vi "getTestTime.vi"(8 "错误输入（无错误）":errorcluster, 11 "startTime":string) -> (0 "错误输出":errorcluster, 3 "timeArray":string[](array[string]))   [LabVIEW 2011]
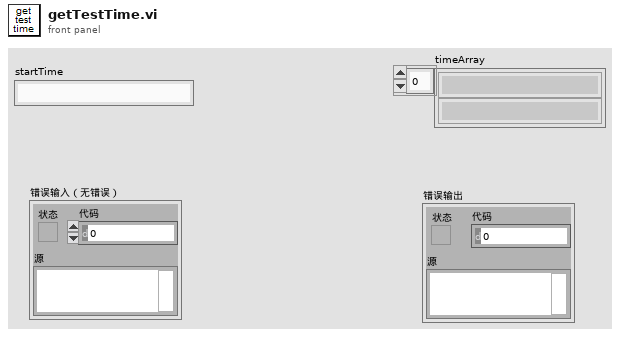
[diagram p1: front panel]
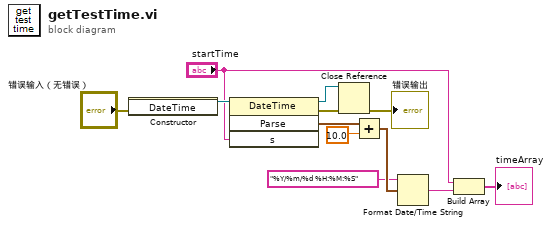
[diagram p0: block diagram]
diagram:
  n1 = constructor class="DateTime"(error in="错误输入（无错误）") -> (reference out=w12:refnum<k24>)  [unwired: 2 in, 2 out]
  n2 = invoke class="DateTime" method="Parse"(reference=w12, "s"="startTime") -> (reference out=w4:refnum<k24>, error out=w3:errorcluster, "Parse"=w11:timestamp)  [unwired: 2 in, 1 out]
  n3 = Close Reference(reference=w4, error in (no error)=w3) -> (error out=→"错误输出":errorcluster)
  n4 = Add(x=w11, y=10.0) -> (x+y=w9:timestamp)
  n5 = Format Date/Time String(time format string (%c)="%Y/%m/%d %H:%M:%S" ("时间格式字符串(%c)"), seconds (now)=w9) -> (date/time string=w6:string)  [unwired: 1 in]
  n6 = Build Array("startTime", w6) -> (→"timeArray":string[])
